vi "Set Denstinations Count.vi"(7 "Destination Count":i32, 8 "error in (no error)":errorcluster, 11 "BuildSpect in":refnum<vi>) -> (0 "error out":errorcluster, 3 "BuildSpec out":refnum<vi>)   [LabVIEW 2019, in "Project Sync Tools.lvclass"]
uses:
  Project Sync Tools.lvclass
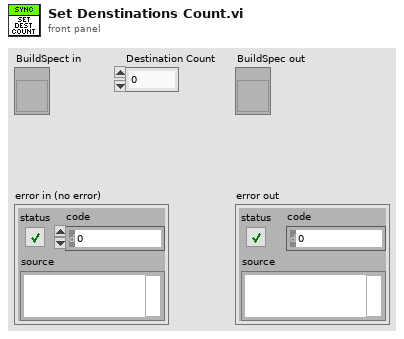
[diagram p1: front panel]
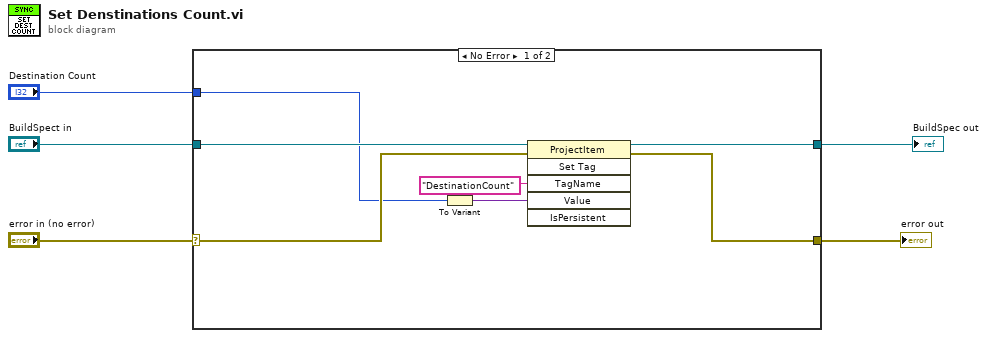
[diagram p0: block diagram]
diagram:
  n1 = case shown="No Error" "error in (no error)" {
    selector: "error in (no error)" -> [w9 w13]
    tunnel: [w12 w13] -> w5
    tunnel: [w11 w14] -> w4
    tunnel: "BuildSpect in" -> [w10 w14]
    tunnel: "Destination Count" -> [w6 _]
    frame No Error {
      n2 = To Variant(anything=w6) -> (Variant=w8:variant)
      n3 = invoke class="ProjectItem" method="Set Tag"(reference=w10, error in=w9, "TagName"="DestinationCount" ("Tag Name"), "Value"=w8) -> (reference out=w11:refnum<vi>, error out=w12:errorcluster)  [unwired: 2 in, 4 out]
    }
    frame Error {
    }
  }
  "error out" <- w5
  "BuildSpec out" <- w4
